vi "findIndirectPath.vi"(8 "error in (no error)":errorcluster, 10 "goal platform":i32, 11 "start platform":i32) -> (0 "error out":errorcluster, 1 "path axes":i32[](array[numeric]), 2 "intersection \nplatform":dbl[](array[numeric]), 3 "total path":dbl[](array[numeric]), 4 "intersection to goal \ndistance":dbl, 5 "start to intersection distance":dbl)   [LabVIEW 2017]
panel:
  out "intersection to \ngoal path":dbl[](array[numeric])
  out "start to intersection \npath":dbl[](array[numeric])
  out "total length":dbl[][](array[numeric])
  out "intersection to \ngoal distance":dbl[][](array[numeric])
  out "start to intersection \ndistance":dbl[][](array[numeric])
  out "intersection index -\ngoal paths":dbl[][](array[numeric])
  out "intersection index - \nstart paths":dbl[][](array[numeric])
  out "index of goal \nin paths through\ngoal":i32[](array[numeric])
  out "index of start \nin paths through \nstart":i32[](array[numeric])
  out "paths through start":dbl[][](array[numeric])
  out "paths through goal":dbl[][](array[numeric])
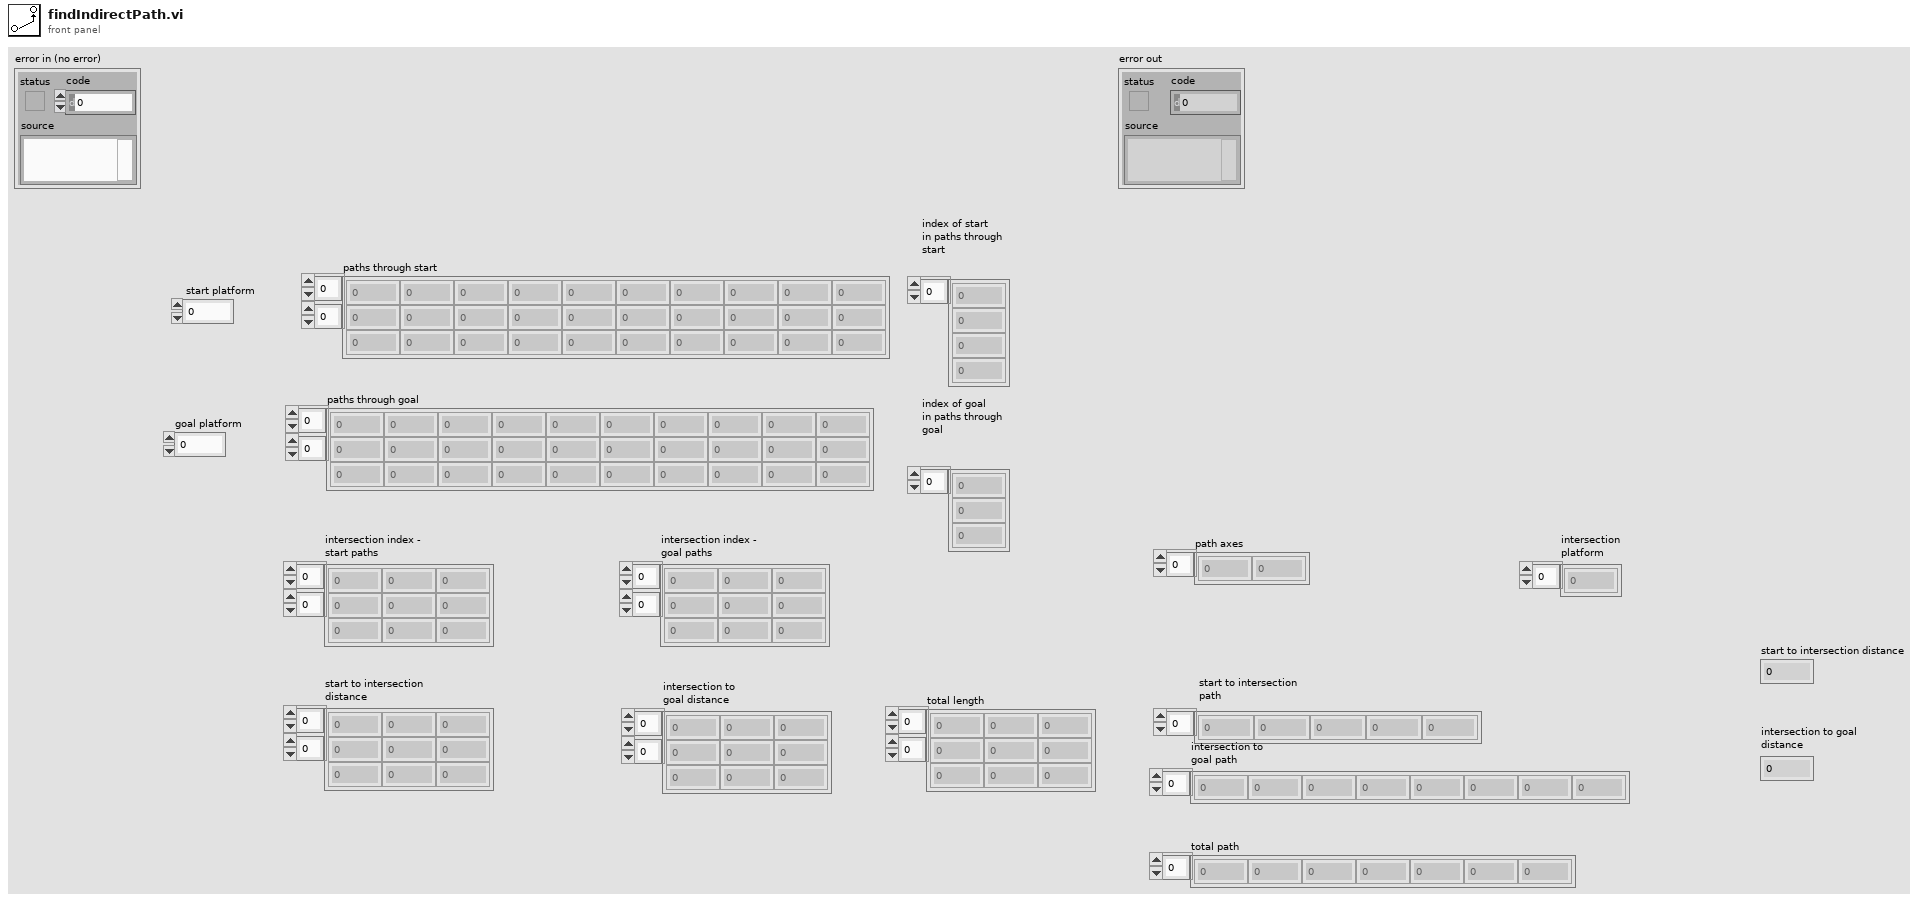
[diagram p1: front panel]
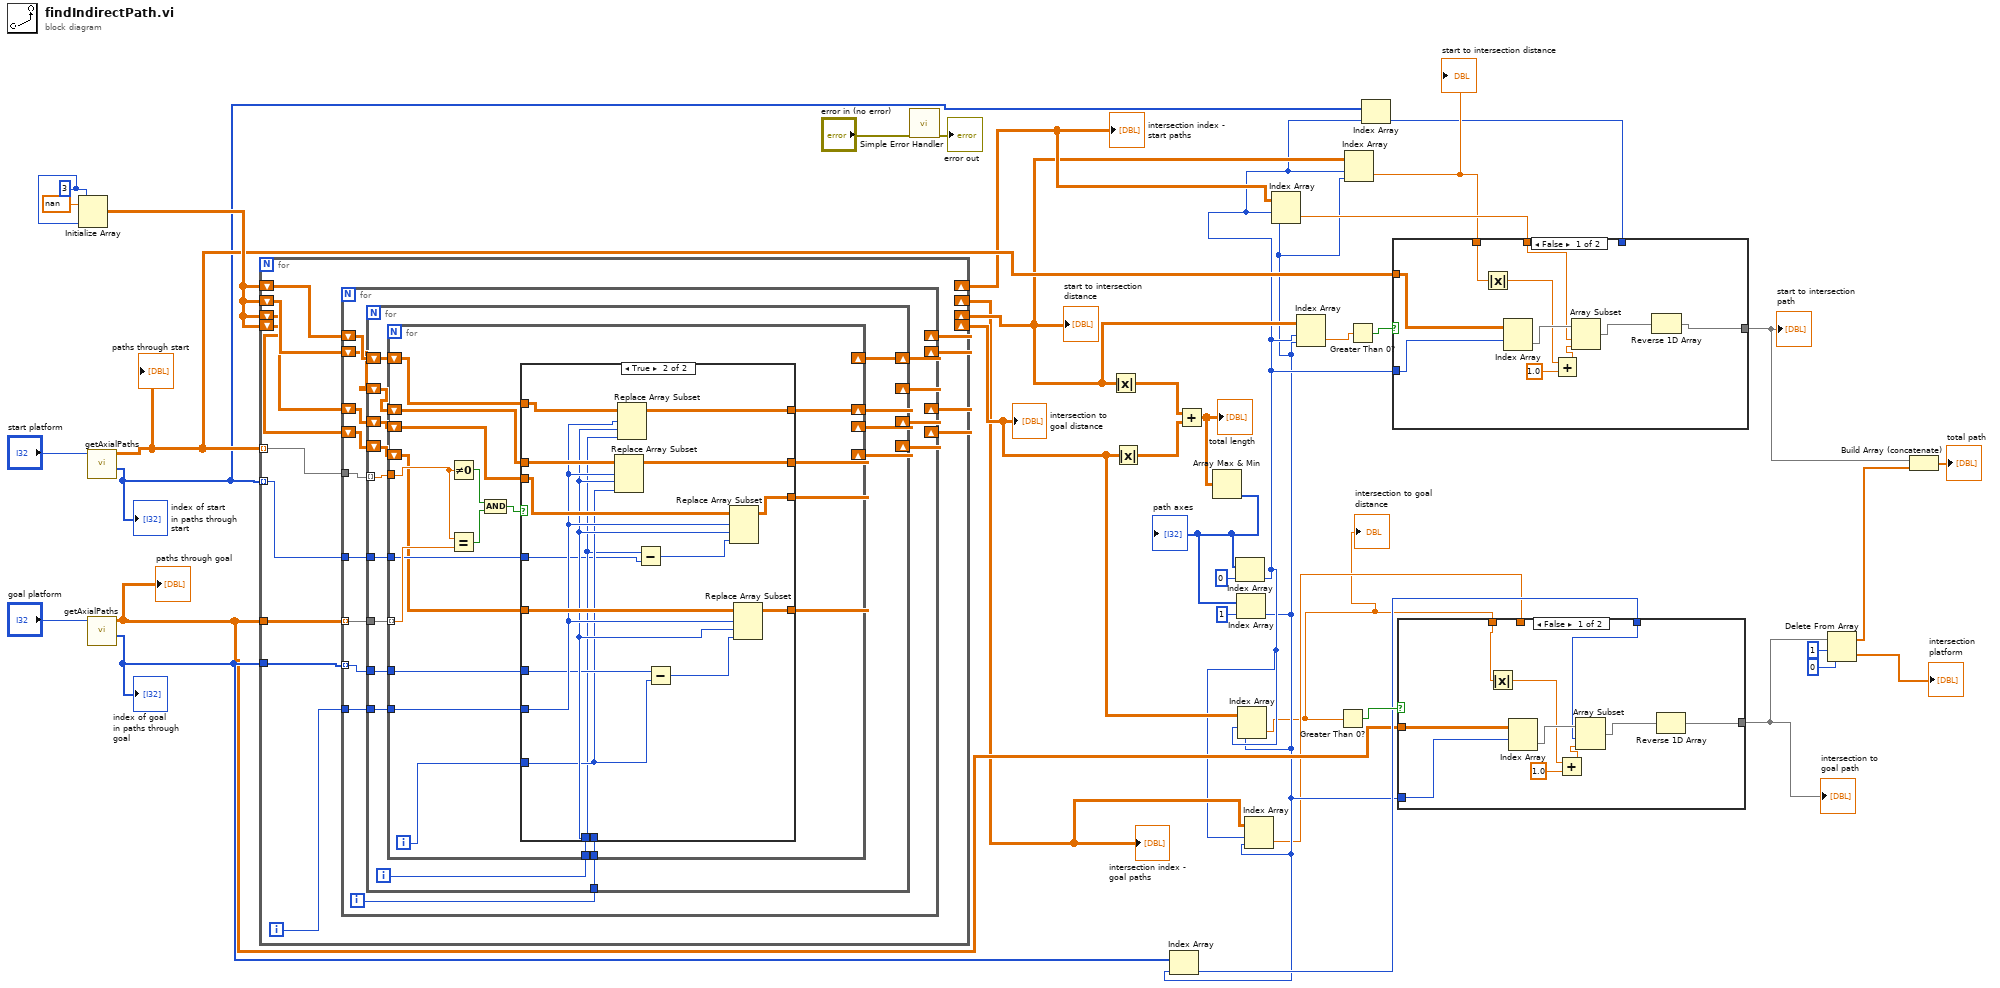
[diagram p0: block diagram]
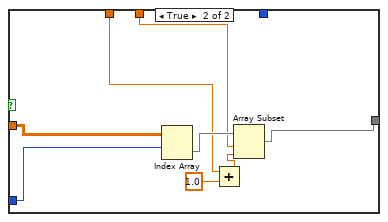
[diagram p2: hidden frame]
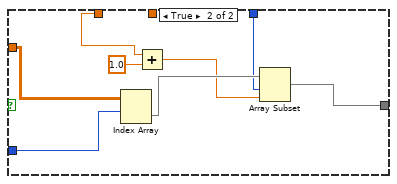
[diagram p3: hidden frame]
diagram:
  w34 = 3 ("dimension size")
  n1 = Initialize Array(nan ("element"), w34, w34) -> (w33:dbl[][])
  n2 = call "getAxialPaths.vi"("platform"="start platform") -> ("platform indices"=w17:i32[], "paths through start"=w22:dbl[][])  [unwired: 9 in]
  "paths through start" <- w22
  "index of start \nin paths through \nstart" <- w17
  n3 = call "getAxialPaths.vi"("platform"="goal platform") -> ("platform indices"=w15:i32[], "paths through start"=w13:dbl[][])  [unwired: 9 in]
  "paths through goal" <- w13
  "index of goal \nin paths through\ngoal" <- w15
  n4 = for {
    tunnel: w22 -> [w51] mode=indexing
    shift-right: [w47] -> w21
    shift-left: w33 -> [w50]
    shift-right: [w45] -> w12
    shift-left: w33 -> [w46]
    shift-right: [w42] -> w19
    shift-left: w33 -> [w44]
    shift-right: [w40] -> w26
    shift-left: w33 -> [w41]
    tunnel: w13 -> [w52]
    tunnel: w17 -> [w43] mode=indexing
    tunnel: w15 -> [w49]
    i -> [w48]
    n5 = for {
      tunnel: w52 -> [w65] mode=indexing
      tunnel: w51 -> [w66]
      shift-right: [w61] -> w47
      shift-left: w50 -> [w64]
      tunnel: w49 -> [w54] mode=indexing
      tunnel: w48 -> [w63]
      shift-right: [w59] -> w45
      shift-left: w46 -> [w60]
      shift-right: [w56] -> w42
      shift-left: w44 -> [w58]
      tunnel: w43 -> [w57]
      shift-right: [w53] -> w40
      shift-left: w41 -> [w55]
      i -> [w62]
      n6 = for {
        tunnel: w66 -> [w81] mode=indexing
        tunnel: w65 -> [w80]
        shift-right: [w75] -> w61
        shift-left: w64 -> [w79]
        tunnel: w63 -> [w78]
        tunnel: w62 -> [w77]
        shift-right: [w73] -> w59
        shift-left: w60 -> [w74]
        shift-right: [w70] -> w56
        shift-left: w58 -> [w72]
        tunnel: w57 -> [w71]
        shift-right: [w67] -> w53
        shift-left: w55 -> [w69]
        tunnel: w54 -> [w68]
        i -> [w76]
        n7 = for {
          tunnel: w81 -> [w100]
          tunnel: w80 -> [w99] mode=indexing
          shift-right: [w91] -> w75
          shift-left: w79 -> [w95]
          tunnel: w78 -> [w94]
          tunnel: w77 -> [w93]
          tunnel: w76 -> [w92]
          shift-right: [w88] -> w73
          shift-left: w74 -> [w90]
          shift-right: [w85] -> w70
          shift-left: w72 -> [w87]
          tunnel: w71 -> [w86]
          shift-right: [w82] -> w67
          shift-left: w69 -> [w84]
          tunnel: w68 -> [w83]
          i -> [w89]
          n8 = Not Equal To 0?(x=w100) -> (x != 0?=w97:bool)
          n9 = Equal?(x=w100, y=w99) -> (x = y?=w98:bool)
          n10 = And(x=w97, y=w98) -> (x .and. y?=w96:bool)
          n11 = case shown="True" w96 {
            tunnel: w95 -> [w104 w120]
            tunnel: w94 -> [_ w112]
            tunnel: w93 -> [_ w111]
            tunnel: w92 -> [_ w106]
            tunnel: [w104 w119] -> w91
            tunnel: w90 -> [w103 w118]
            tunnel: w89 -> [_ w109]
            tunnel: [w103 w117] -> w88
            tunnel: w87 -> [w102 w116]
            tunnel: w86 -> [_ w105]
            tunnel: [w102 w114] -> w85
            tunnel: w84 -> [w101 w113]
            tunnel: w83 -> [_ w110]
            tunnel: [w101 w107] -> w82
            frame False {
            }
            frame True {
              n12 = Replace Array Subset(array=w118, new element=w109, index (row)=w112, index (col)=w111) -> (w117:dbl[][])
              n13 = Replace Array Subset(array=w120, new element=w106, index (row)=w112, index (col)=w111) -> (w119:dbl[][])
              n14 = Subtract(x=w106, y=w105) -> (x-y=w115:i32)
              n15 = Subtract(x=w110, y=w109) -> (x-y=w108:i32)
              n16 = Replace Array Subset(array=w116, new element=w115, index (row)=w112, index (col)=w111) -> (w114:dbl[][])
              n17 = Replace Array Subset(array=w113, new element=w108, index (row)=w112, index (col)=w111) -> (w107:dbl[][])
            }
          }
        }
      }
    }
  }
  "intersection index - \nstart paths" <- w21
  "intersection index -\ngoal paths" <- w12
  "start to intersection \ndistance" <- w19
  "intersection to \ngoal distance" <- w26
  n18 = call <vilib>:"Simple Error Handler.vi"("error in (no error)"="error in (no error)") -> ("error out"=→"error out":errorcluster)  [unwired: 4 in, 4 out]
  n19 = Absolute Value(x=w19) -> (abs(x)=w32:dbl[][])
  n20 = Absolute Value(x=w26) -> (abs(x)=w31:dbl[][])
  n21 = Add(x=w32, y=w31) -> (x+y=w30:dbl[][])
  "total length" <- w30
  n22 = Array Max & Min(array=w30) -> (min index (indices)=w28:i32[])  [unwired: 3 out]
  "path axes" <- w28
  n23 = Index Array(array=w28, index=0) -> (element=w11:i32)
  n24 = Index Array(array=w28, index=1) -> (element=w10:i32)
  n25 = Index Array(array=w15, index=w10) -> (element=w14:i32)
  n26 = Index Array(array=w26, index (row)=w11, index (col)=w10) -> (element=w1:dbl)
  "intersection to goal \ndistance" <- w1
  n27 = Index Array(array=w12, index (row)=w11, index (col)=w10) -> (element=w9:dbl)
  n28 = Index Array(array=w21, index (row)=w11, index (col)=w10) -> (element=w20:dbl)
  n29 = Index Array(array=w19, index (row)=w11, index (col)=w10) -> (element=w25:dbl)
  n30 = Greater Than 0?(x=w1) -> (x > 0?=w23:bool)
  n31 = Index Array(array=w19, index (row)=w11, index (col)=w10) -> (element=w18:dbl)
  "start to intersection distance" <- w18
  n32 = Greater Than 0?(x=w25) -> (x > 0?=w24:bool)
  n33 = Index Array(array=w17, index=w11) -> (element=w16:i32)
  n34 = case shown="False" w24 {
    tunnel: w22 -> [w130 w138]
    tunnel: w11 -> [w129 w137]
    tunnel: w20 -> [w126 _]
    tunnel: w18 -> [w127 w133]
    tunnel: [w122 w135] -> w8
    tunnel: w16 -> [_ w134]
    frame False {
      n35 = Absolute Value(x=w127) -> (abs(x)=w125:dbl)
      n36 = Index Array(array=w130, index (row)=w129) -> (element=w128:dbl[])  [unwired: 1 in]
      n37 = Add(x=w125, y=1.0) -> (x+y=w123:dbl)
      n38 = Array Subset(array=w128, index=w126, length=w123) -> (w121:dbl[])
      n39 = Reverse 1D Array(array=w121) -> (reversed array=w122:dbl[])
    }
    frame True {
      n40 = Index Array(array=w138, index (row)=w137) -> (element=w136:dbl[])  [unwired: 1 in]
      n41 = Add(x=w133, y=1.0) -> (x+y=w132:dbl)
      n42 = Array Subset(array=w136, index=w134, length=w132) -> (w135:dbl[])
    }
  }
  "start to intersection \npath" <- w8
  n43 = case shown="False" w23 {
    tunnel: w14 -> [w139 _]
    tunnel: w13 -> [w143 w152]
    tunnel: w10 -> [w142 w151]
    tunnel: w1 -> [w141 w153]
    tunnel: w9 -> [_ w149]
    tunnel: [w140 w150] -> w7
    frame False {
      n44 = Absolute Value(x=w141) -> (abs(x)=w147:dbl)
      n45 = Index Array(array=w143, index (row)=w142) -> (element=w148:dbl[])  [unwired: 1 in]
      n46 = Add(x=w147, y=1.0) -> (x+y=w145:dbl)
      n47 = Array Subset(array=w148, index=w139, length=w145) -> (w144:dbl[])
      n48 = Reverse 1D Array(array=w144) -> (reversed array=w140:dbl[])
    }
    frame True {
      n49 = Index Array(array=w152, index (row)=w151) -> (element=w156:dbl[])  [unwired: 1 in]
      n50 = Add(x=w153, y=1.0) -> (x+y=w154:dbl)
      n51 = Array Subset(array=w156, index=w149, length=w154) -> (w150:dbl[])
    }
  }
  "intersection to \ngoal path" <- w7
  n52 = Delete From Array(array=w7, length=1, index=0) -> (deleted portion=→"intersection \nplatform":dbl[], array with subset deleted=w4:dbl[])
  n53 = Build Array (concatenate)(w8, w4) -> (→"total path":dbl[])
